vi "ErrorHandler.vi"(8 "error in (no error)":errorcluster, 10 "Interactive":bool=TRUE) -> (0 "error out":errorcluster, 3 "Error":bool)   [LabVIEW 2014]
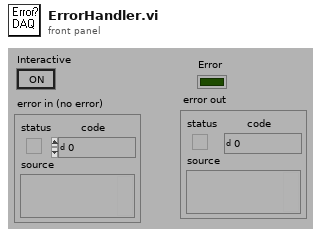
[diagram p1: front panel]
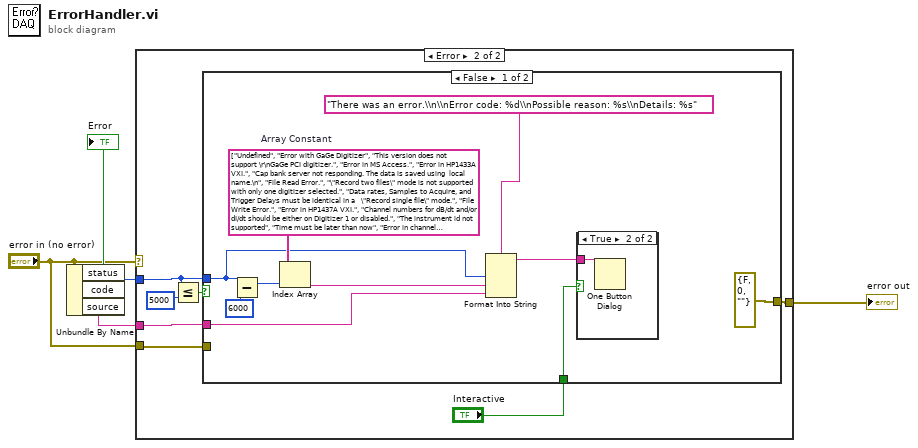
[diagram p0: block diagram]
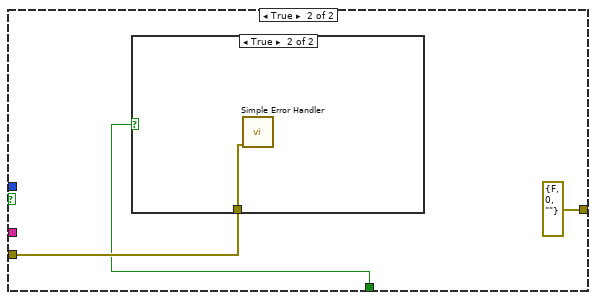
[diagram p4: hidden frame]
diagram:
  n1 = Unbundle By Name("error in (no error)") -> ("status"=→"Error":bool, "code"=w4:i32, "source"=w2:string)
  n2 = case shown="Error" "error in (no error)" {
    tunnel: w4 -> [_ w9]
    tunnel: "error in (no error)" -> [w6 w7]
    tunnel: [w6 w12] -> w3
    tunnel: w2 -> [_ w13]
    frame No Error {
    }
    frame Error {
      n3 = Less Or Equal?(x=w9, y=5000 ("x")) -> (x <= y?=w8:bool)
      n4 = case shown="False" w8 {
        tunnel: w9 -> [w19 _]
        tunnel: w13 -> [w14 _]
        tunnel: [errorcluster {"status"=FALSE, "code"=0, "source"=""} ("error in (no error)") errorcluster {"status"=FALSE, "code"=0, "source"=""} ("error in (no error)")] -> w12
        tunnel: "Interactive" -> [w16 w26]
        tunnel: w7 -> [_ w27]
        frame False {
          w21 = string[] ["Undefined", "Error with GaGe Digitizer", "This version does not support \r\nGaGe PCI digitizer.", "Error in MS Access.", "Error in HP1433A VXI.", "Cap bank server not responding. The data is saved using  local name.\n", "File Read Error.", "\"Record two files\" mode is not supported with only one digitizer selected.", "Data rates, Samples to Acquire, and Trigger Delays must be identical in a   \"Record single file\" mode.", "File Write Error.", "Error in HP1437A VXI.", "Channel numbers for dB/dt and/or dI/dt should be either on Digitizer 1 or disabled.", "The instrument id not supported", "Time must be later than now", "Error in channel integration"]  # Array Constant
          n5 = Subtract(x=w19, y=6000) -> (x-y=w22:i32)
          n6 = Index Array(array=w21, index=w22) -> (element=w15:string)
          n7 = Format Into String(format string="There was an error.\\n\\nError code: %d\\nPossible reason: %s\\nDetails: %s" ("Format String"), w19, w15, w14) -> (resulting string=w18:string)  [unwired: 2 in, 1 out]
          n8 = case shown="True" w16 {
            tunnel: w18 -> [_ w24]
            frame False {
            }
            frame True {
              n9 = One Button Dialog(message=w24) -> ()  [unwired: 2 out]
            }
          }
        }
        frame True {
          n10 = case shown="True" w26 {
            tunnel: w27 -> [_ w28]
            frame False {
            }
            frame True {
              n11 = call <vilib>:"Simple Error Handler.vi"("error in (no error)"=w28) -> ()  [unwired: 1 in, 8 out]
            }
          }
        }
      }
    }
  }
  "error out" <- w3
